vi "GetXL_WorkSheetSize.vi"(8 "error in (no error)":errorcluster, 11 "Refnum Cluster in":T1) -> (0 "error out":errorcluster, 1 "# Columns":i32, 2 "# Rows":i32, 3 "Refnum Cluster Out":T1)   [LabVIEW 2017, in "excel_configuration.lvlib"]
uses:
  excel_configuration.lvlib
  b2c6f0f4-7f87-4914-851e-5f335a2ff66f.vi
  8c9d7fcb-4391-4a71-8f51-e2d0cb059e2c.vi
  02983a4b-8016-41e5-a431-1b83200de9b1.vi
  <vilib>/Utility/error.llb/Clear Errors.vi
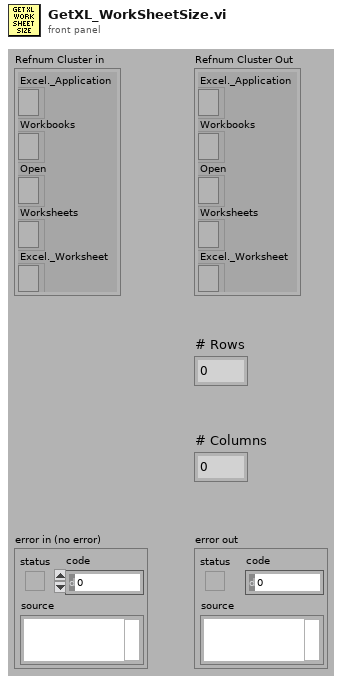
[diagram p1: front panel]
types:
  T1 = cluster{"Excel._Application":refnum<k7>, "Workbooks":refnum<k7>, "Open":refnum<k7>, "Worksheets":refnum<k7>, "Excel._Worksheet":refnum<k7>}
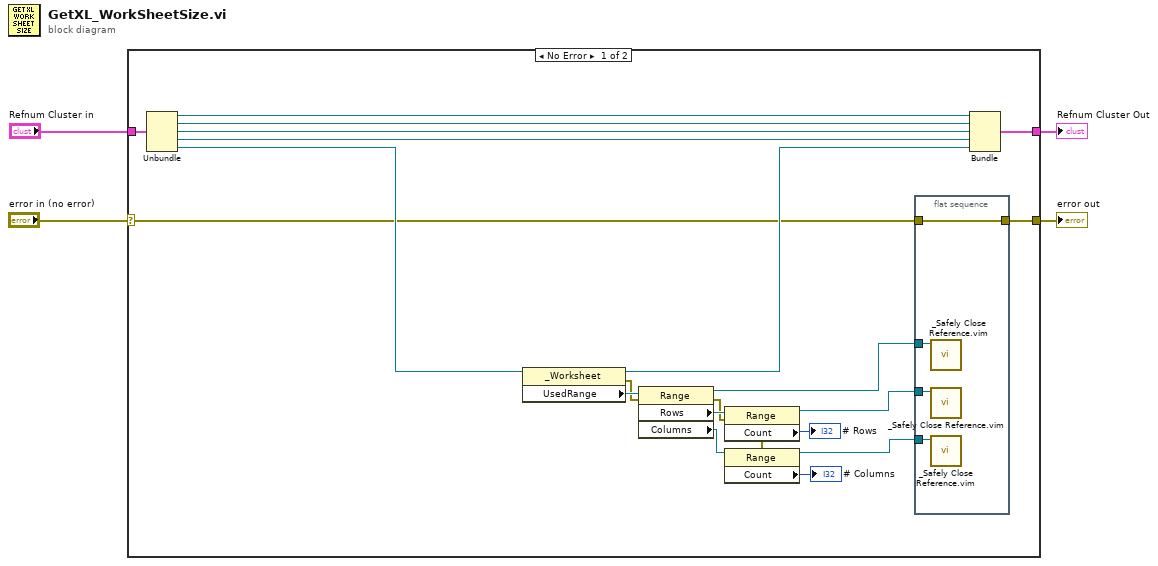
[diagram p0: block diagram]
diagram:
  n1 = case shown="No Error" "error in (no error)" {
    selector: "error in (no error)" -> [w6 w31]
    tunnel: [w22 w30] -> w4
    tunnel: "Refnum Cluster in" -> [w13 w30]
    tunnel: [w5 w31] -> w1
    frame No Error {
      n2 = Unbundle(w13) -> ("Excel._Application"=w23:refnum<k7>, "Workbooks"=w24:refnum<k7>, "Open"=w25:refnum<k7>, "Worksheets"=w10:refnum<k7>, "Excel._Worksheet"=w12:refnum<k7>)
      n3 = property class="_Worksheet"(reference=w12) -> (reference out=w11:refnum<k7>, error out=w19:errorcluster, "UsedRange"=w20:refnum<k7>)  [unwired: 1 in]
      n4 = property class="Range"(reference=w20, error in=w19) -> (reference out=w9:refnum<k7>, error out=w18:errorcluster, "Rows"=w21:refnum<k7>, "Columns"=w16:refnum<k7>)
      n5 = property class="Range"(reference=w21, error in=w18) -> (reference out=w8:refnum<k7>, error out=w14:errorcluster, "Count"=→"# Rows":i32)
      n6 = property class="Range"(reference=w16, error in=w14) -> (reference out=w7:refnum<k7>, "Count"=→"# Columns":i32)  [unwired: 1 out]
      n7 = flat-sequence {
        tunnel: w9 -> [w29]
        tunnel: w8 -> [w28]
        tunnel: w7 -> [w27]
        tunnel: w6 -> [w26]
        tunnel: [w26] -> w5
        frame #0 {
          n8 = call "_Safely Close Reference.vim"("Automation Refnum in"=w29) -> ()  [unwired: 10 in, 1 out]
          n9 = call "_Safely Close Reference.vim"("Automation Refnum in"=w28) -> ()  [unwired: 10 in, 1 out]
          n10 = call "_Safely Close Reference.vim"("Automation Refnum in"=w27) -> ()  [unwired: 10 in, 1 out]
        }
      }
      n11 = Bundle("Excel._Application"=w23, "Workbooks"=w24, "Open"=w25, "Worksheets"=w10, "Excel._Worksheet"=w11) -> (w22:T1)  [unwired: 1 in]
    }
    frame Error {
    }
  }
  "error out" <- w1
  "Refnum Cluster Out" <- w4
